vi "cosmeticPIP.vi"(8 "error in (no error)":errorcluster) -> (0 "error out":errorcluster, 3 "COSMETIC-3, 4":string)   [LabVIEW 2018]
uses:
  Global_usbComm.vi
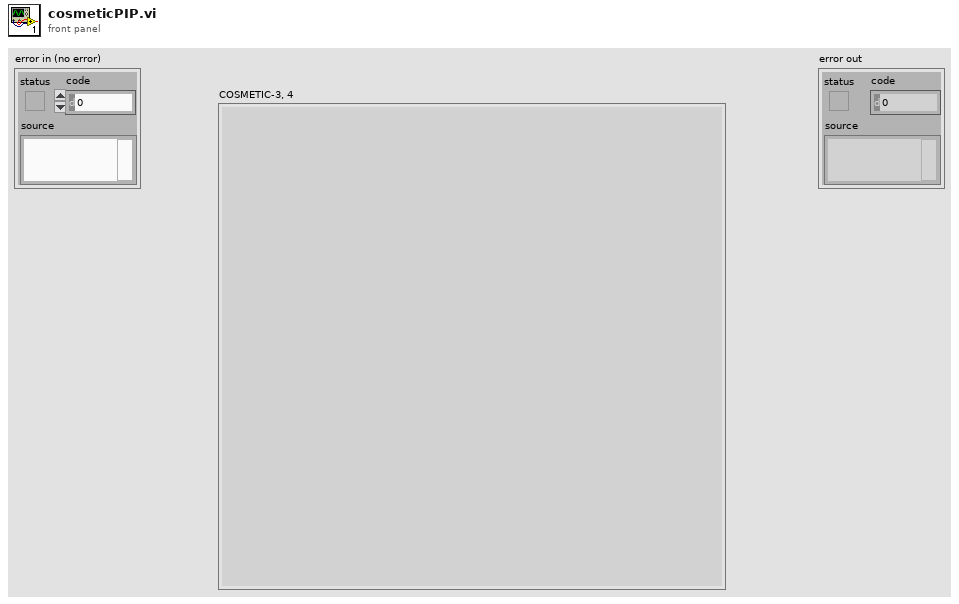
[diagram p1: front panel]
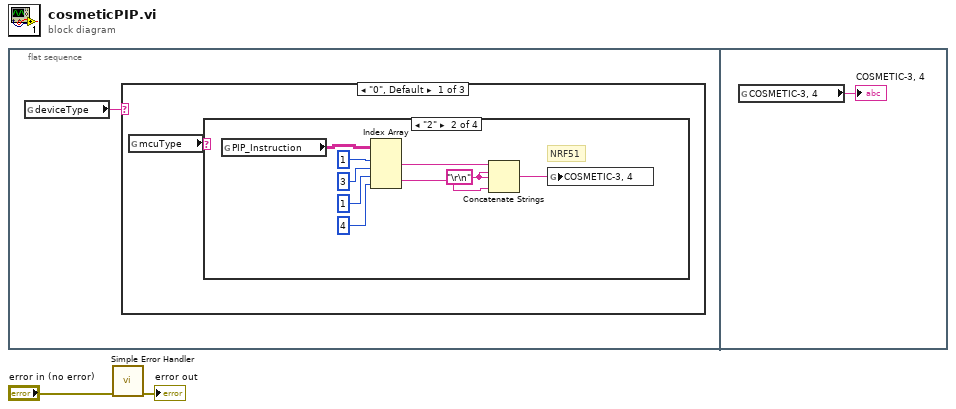
[diagram p0: block diagram]
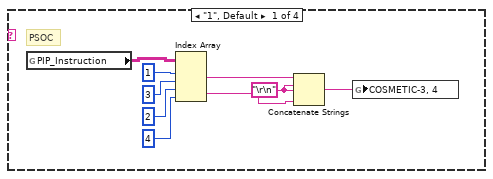
[diagram p2: hidden frame]
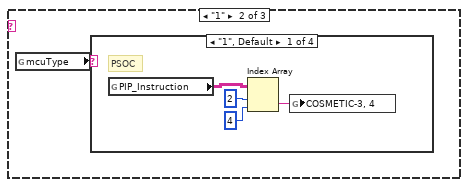
[diagram p5: hidden frame]
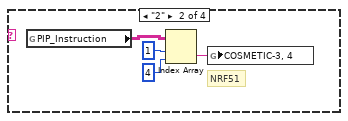
[diagram p6: hidden frame]
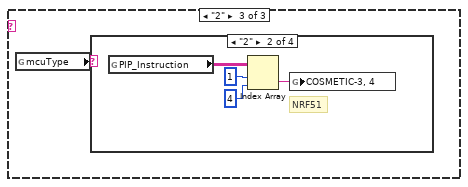
[diagram p9: hidden frame]
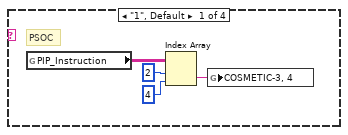
[diagram p10: hidden frame]
diagram:
  n1 = flat-sequence {
    frame #0 {
      n2 = global read "Global_usbComm.vi" "deviceType"() -> (w3:string)
      n3 = case shown="\"0\", Default" w3 {
        frame "0", Default {
          n4 = global read "Global_usbComm.vi" "mcuType"() -> (w4:string)
          n5 = case shown="\"2\"" w4 {
            frame "1", Default {
              w7 = "\r\n"
              # "PSOC"
              n6 = global read "Global_usbComm.vi" "PIP_Instruction"() -> (w13:string[][])
              n7 = Index Array(array=w13, index (row) #1=1 ("index (row)"), index (col) #1=3 ("disabled index (col)"), index (row) #2=2 ("index (row)"), index (col) #2=4 ("disabled index (col)")) -> (element #1=w8:string, element #2=w6:string)
              n8 = Concatenate Strings(w8, w7, w7, w6) -> (w5:string)
              n9 = global write "Global_usbComm.vi" "COSMETIC-3, 4"(w5) -> ()
            }
            frame "2" {
              w16 = "\r\n"
              # "NRF51"
              n10 = global read "Global_usbComm.vi" "PIP_Instruction"() -> (w22:string[][])
              n11 = Index Array(array=w22, index (row) #1=1 ("index (row)"), index (col) #1=3 ("disabled index (col)"), index (row) #2=1 ("index (row)"), index (col) #2=4 ("disabled index (col)")) -> (element #1=w17:string, element #2=w15:string)
              n12 = Concatenate Strings(w17, w16, w16, w15) -> (w14:string)
              n13 = global write "Global_usbComm.vi" "COSMETIC-3, 4"(w14) -> ()
            }
            frame "3" {
              # "RENESAS"
            }
            frame "4" {
              # "XILOG"
            }
          }
        }
        frame "1" {
          n14 = global read "Global_usbComm.vi" "mcuType"() -> (w23:string)
          n15 = case shown="\"1\", Default" w23 {
            frame "1", Default {
              # "PSOC"
              n16 = global read "Global_usbComm.vi" "PIP_Instruction"() -> (w27:string[][])
              n17 = Index Array(array=w27, index (row)=2, index (col)=4 ("disabled index (col)")) -> (element=w24:string)
              n18 = global write "Global_usbComm.vi" "COSMETIC-3, 4"(w24) -> ()
            }
            frame "2" {
              # "NRF51"
              n19 = global read "Global_usbComm.vi" "PIP_Instruction"() -> (w31:string[][])
              n20 = Index Array(array=w31, index (row)=1, index (col)=4 ("disabled index (col)")) -> (element=w28:string)
              n21 = global write "Global_usbComm.vi" "COSMETIC-3, 4"(w28) -> ()
            }
            frame "3" {
              # "RENESAS"
            }
            frame "4" {
              # "XILOG"
            }
          }
        }
        frame "2" {
          n22 = global read "Global_usbComm.vi" "mcuType"() -> (w32:string)
          n23 = case shown="\"2\"" w32 {
            frame "1", Default {
              # "PSOC"
              n24 = global read "Global_usbComm.vi" "PIP_Instruction"() -> (w36:string[][])
              n25 = Index Array(array=w36, index (row)=2, index (col)=4 ("disabled index (col)")) -> (element=w33:string)
              n26 = global write "Global_usbComm.vi" "COSMETIC-3, 4"(w33) -> ()
            }
            frame "2" {
              # "NRF51"
              n27 = global read "Global_usbComm.vi" "PIP_Instruction"() -> (w40:string[][])
              n28 = Index Array(array=w40, index (row)=1, index (col)=4 ("disabled index (col)")) -> (element=w37:string)
              n29 = global write "Global_usbComm.vi" "COSMETIC-3, 4"(w37) -> ()
            }
            frame "3" {
              # "RENESAS"
            }
            frame "4" {
              # "XILOG"
            }
          }
        }
      }
    }
    frame #1 {
      n30 = global read "Global_usbComm.vi" "COSMETIC-3, 4"() -> (→"COSMETIC-3, 4":string)
    }
  }
  n31 = call <vilib>:"Simple Error Handler.vi"("error in (no error)"="error in (no error)") -> ("error out"=→"error out":errorcluster)  [unwired: 4 in, 4 out]
